vi "在表格中插入空白列.vi"(10 "插入列位置":i32[](array[numeric]), 11 "表格输入":string[][](array[string])) -> (3 "表格输出":string[][](array[string]))   [LabVIEW 2014, in "表格.lvlib"]
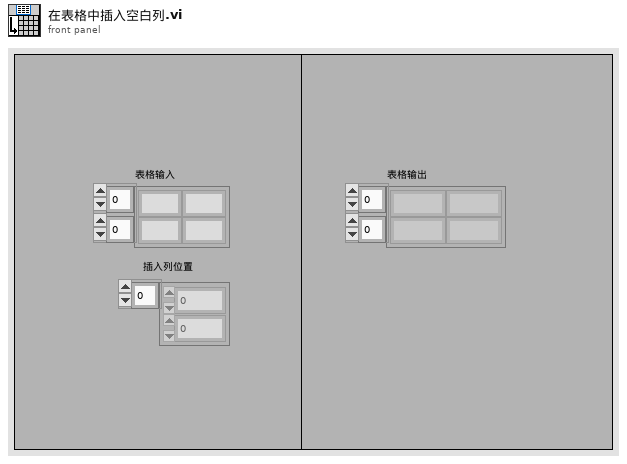
[diagram p1: front panel]
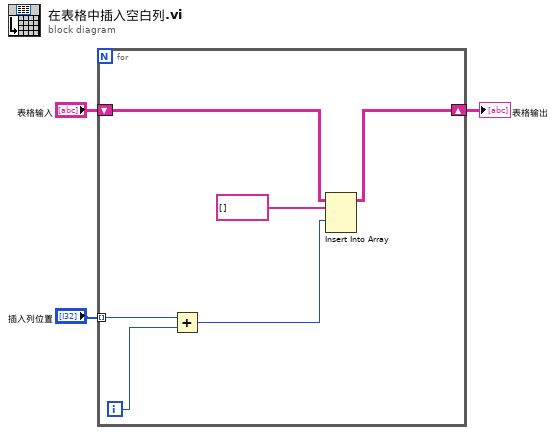
[diagram p0: block diagram]
diagram:
  n1 = for {
    shift-right: [w9] -> w3
    shift-left: "表格输入" -> [w8]
    tunnel: "插入列位置" -> [w5] mode=indexing
    i -> [w6]
    n2 = Add(x=w5, y=w6) -> (x+y=w4:i32)
    n3 = Insert Into Array(array=w8, index (col)=w4, new element=string[] [] ("新元素/子数组")) -> (w9:string[][])  [unwired: 1 in]
  }
  "表格输出" <- w3
